vi "Spectrometer - Standalone.vi"() -> ()   [LabVIEW 2014]
uses:
  Laser Settings.ctl
  Laser.ctl
  Filter.ctl
  Grating Detector Settings.ctl
  Grating.ctl
  Detector.ctl
  Acquisition Settings.ctl
  support/Instrument Status.ctl
  Spectrometer Config.ctl
  Spectrometer Refnum.ctl
  Measurements/Plot Data/Optical Spectrum Plot Refnum.ctl
  support/User Event - Stop/User Event - Stop.lvlib
  support/Message Queue/Message Queue.lvlib
panel:
  out "Instrument Status":T1
  out "Status Log":string
  in  "Laser Settings":T2={"Laser Wavelength"=enum."633 nm", "Neutral Density Filter"=enum."1%"}
  in  "Spectrometer Settings":T5={"Confocal Hole Size (µm)"=150.0, "Grating"=1, "Detector"=enum."InGaAs Array"} {"Grating" items=["1800 l/mm", "150 l/mm"]}
  in  "Acquisition Settings":T8={"Acquisition Mode"=enum."Single Window", "Spectal Position (nm)"=480.0, "From (nm)"=632.0, "To (nm)"=1000.0, "Integration Time (s)"=3.0, "Number of Accumulations"=3, "AutoScanning"=FALSE, "Spike Removal"=FALSE}
  in  "Optical Spectrum":enum32{"Energy", "Wavelength", "Raman Shift"}(tab)
  out "Optical Spectrum vs Energy":cluster{"data":dbl[], "data":dbl[]}(graph)
  out "Optical Spectrum vs Wavelength":cluster{"data":dbl[], "data":dbl[]}(graph)
  out "Optical Spectrum vs Raman Shift":cluster{"data":dbl[], "data":dbl[]}(graph)
  in  "Optical Spectrometer - Save Measurement":bool
  in  "Optical Spectrometer - Measure":bool
  out "Detector Temperature":dbl
  in  "Use Labram HR":bool=TRUE
  out "Last Operation":string
  in  "Exit":bool
  # "LICENSED MATERIALS – PROPERTY OF IBM\nCopyright IBM Corp. 2016,\nALL RIGHTS RESERVED"
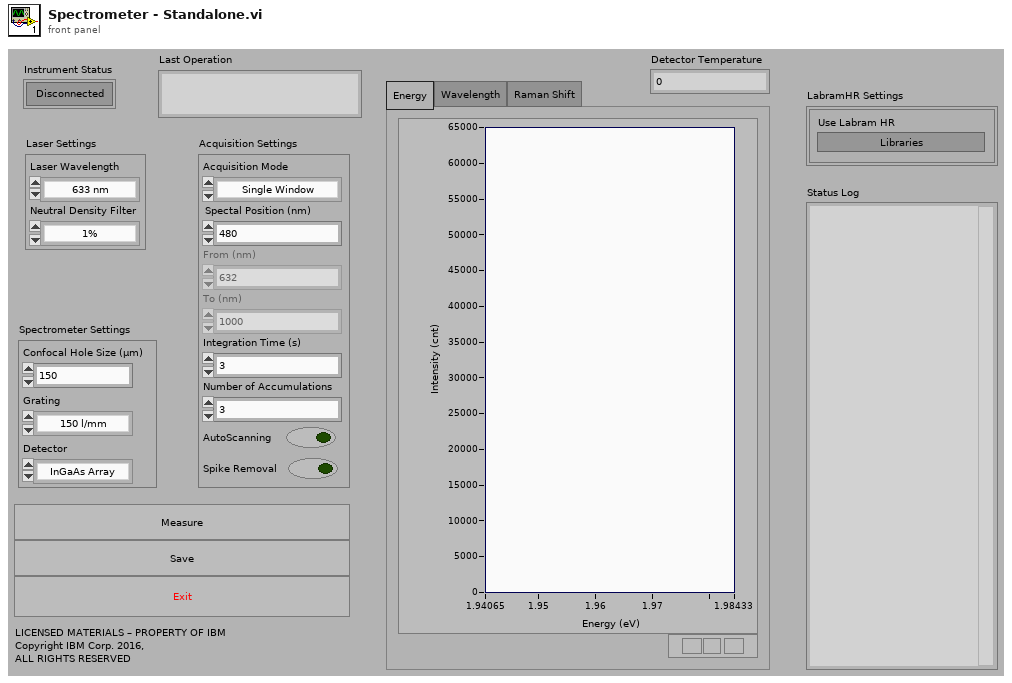
[diagram p1: front panel]
types:
  T1 = typedef "Instrument Status.ctl" = bool
  T2 = typedef "Laser Settings.ctl" = cluster{"Laser Wavelength":T3, "Neutral Density Filter":T4}
  T3 = typedef "Laser.ctl" = enum16{"633 nm", "784 nm", "532 nm", "365 nm"}
  T4 = typedef "Filter.ctl" = enum16{"100%", "50%", "25%", "10%", "1%", "0.1%", "0.01%"}
  T5 = typedef "Grating Detector Settings.ctl" = cluster{"Confocal Hole Size (µm)":dbl, "Grating":T6, "Detector":T7}
  T6 = typedef "Grating.ctl" = u16
  T7 = typedef "Detector.ctl" = enum16{"InGaAs Array", "Silicon CCD"}
  T8 = typedef "Acquisition Settings.ctl" = cluster{"Acquisition Mode":enum16{"Single Window", "Multi-Window"}, "Spectal Position (nm)":dbl, "From (nm)":dbl, "To (nm)":dbl, "Integration Time (s)":dbl, "Number of Accumulations":i32, "AutoScanning":bool, "Spike Removal":bool}
  T9 = typedef "Message Queue.lvlib/All Message Queues.ctl" = cluster{"Message Handler Loop":refnum<queue>, "Parameter Analyzer":refnum<queue>, "Switching Matrix":refnum<queue>, "Stress Control":refnum<queue>, "Optical Spectrometer":refnum<queue>, "Switches & Mirrors":refnum<queue>, "Camera":refnum<queue>, "XYZ Stage":refnum<queue>, "AutoFocus":refnum<queue>, "Optoelectronic":refnum<queue>, "Save Data":refnum<queue>, "Plot Data":refnum<queue>, "Instrument Sequence":refnum<queue>, "Strain Measurement":refnum<queue>}
  T10 = typedef "Notifiers.ctl" = cluster{"Message Handler Loop":T11, "Parameter Analyzer":T12, "Switching Matrix":T13, "Stress Control":T14, "Optical Spectrometer":T15, "Switches & Mirrors":T16, "Camera":T17, "XYZ Stage":T18, "AutoFocus":T19, "Optoelectronic":T20, "Save Data":T21, "Plot Data":T21, "Instrument Sequence":T22, "Strain Measurement":cluster{"Status":refnum<notifier>, "Exit":refnum<notifier>, "Ready":refnum<notifier>}}
  T11 = typedef "Message Handler Loop Notifiers.ctl" = cluster{"Status":refnum<notifier>, "Instrument Data":refnum<notifier>, "Exit":refnum<notifier>, "Ready":refnum<notifier>}
  T12 = typedef "Parameter Analyzer Notifiers.ctl" = cluster{"Status":refnum<notifier>, "Instrument Data":refnum<notifier>, "Measurement":refnum<notifier>, "Exit":refnum<notifier>, "Ready":refnum<notifier>}
  T13 = typedef "Switching Matrix Notifiers.ctl" = cluster{"Status":refnum<notifier>, "Instrument Data":refnum<notifier>, "Measurement":refnum<notifier>, "Exit":refnum<notifier>, "Ready":refnum<notifier>}
  T14 = typedef "StressControl Notifiers.ctl" = cluster{"Status":refnum<notifier>, "Instrument Data":refnum<notifier>, "Measurement":refnum<notifier>, "Exit":refnum<notifier>, "Ready":refnum<notifier>}
  T15 = typedef "Spectrometer Notifiers.ctl" = cluster{"Status":refnum<notifier>, "Instrument Data":refnum<notifier>, "Measurement":refnum<notifier>, "Exit":refnum<notifier>, "Ready":refnum<notifier>}
  T16 = typedef "SwitchesMirrors Notifiers.ctl" = cluster{"Status":refnum<notifier>, "Instrument Data":refnum<notifier>, "Exit":refnum<notifier>, "Ready":refnum<notifier>}
  T17 = typedef "Camera Notifiers.ctl" = cluster{"Status":refnum<notifier>, "Instrument Data":refnum<notifier>, "Measurement":refnum<notifier>, "Exit":refnum<notifier>, "Ready":refnum<notifier>}
  T18 = typedef "XYZ Notifications.ctl" = cluster{"Status":refnum<notifier>, "Instrument Data":refnum<notifier>, "Measurement":refnum<notifier>, "Exit":refnum<notifier>, "Ready":refnum<notifier>}
  T19 = typedef "Autofocus Notifiers.ctl" = cluster{"Status":refnum<notifier>, "Instrument Data":refnum<notifier>, "Measurement":refnum<notifier>, "Exit":refnum<notifier>, "Ready":refnum<notifier>}
  T20 = typedef "Optoelectronic Notifiers.ctl" = cluster{"Status":refnum<notifier>, "Instrument Data":refnum<notifier>, "Measurement":refnum<notifier>, "Exit":refnum<notifier>, "Ready":refnum<notifier>}
  T21 = typedef "SaveData Notifiers.ctl" = cluster{"Status":refnum<notifier>, "Exit":refnum<notifier>, "Ready":refnum<notifier>}
  T22 = typedef "Instrument Sequence Notifiers.ctl" = cluster{"Status":refnum<notifier>, "Instrument Data":refnum<notifier>, "Measurement":refnum<notifier>, "Exit":refnum<notifier>, "Ready":refnum<notifier>}
  T23 = typedef "Configuration.ctl" = cluster{"Parameter Analizer":T24, "Switching Matrix":T32, "Stress Control":T33, "Optical Spectrometer":T34, "Switches & Mirrors":T35, "Camera":T37, "XYZ Stage":T39, "AutoFocus":T43, "Sava Data":T46, "PlotData":T51, "Instrument Sequence":T57, "Strain Measurement":T58}
  T24 = typedef "Parameter Analyzer Config.ctl" = cluster{"Parameter Analyzer VISA Session":refnum<visa-resource-name>, "Sweeping Time Parameters":T25, "Acquisition Mode":enum32{"Sweeping Mode", "Sampling Mode"}, "Status Polling Time (ms)":u32, "Comment":string, "SMU 1 - Sweeping":T26, "SMU 2 - Sweeping":T26, "SMU 3 - Sweeping":T26, "SMU 4 - Sweeping":T26, "Sweep Spacing":T27, "Range":T28, "SMU1 - Sampling":T29, "SMU2 - Sampling":T29, "SMU3 - Sampling":T29, "SMU4 - Sampling":T29, "Sampling Time Parameters":T30, "Stop Condition":T31}
  T25 = typedef "Parameter Analyzer Integration Parameters.ctl" = cluster{"Integration Time":u32, "Short Integration Time (s)":dbl, "Long Integration Time (s)":dbl, "Wait Time Parameter":dbl}
  T26 = typedef "Parameter Analyzer SMU Sweeping.ctl" = cluster{"Start / Offset":dbl, "Stop / Ratio":dbl, "Step \n(linear only)":dbl, "Compliance":dbl, "Power \nCompliance":dbl, "Mode":u32, "Function":i32, "Sweep Mode":bool}
  T27 = typedef "Parameter Analyzer Sweep Spacing.ctl" = u16
  T28 = typedef "Parameter Analyzer SMU Range.ctl" = u16
  T29 = typedef "Parameter Analyzer SMU Sampling.ctl" = cluster{"Source":dbl, "Compliance":dbl, "Mode":u32, "Function":bool}
  T30 = typedef "Parameter Analyzer Sampling Parameters.ctl" = cluster{"Initial Interval (s)":dbl, "Number of Samples":i32, "Total Sampling Time (s)":dbl, "Hold Time (s)":dbl, "Sampling Mode":i32, "Sampling Time":i32}
  T31 = typedef "Parameter Analyzer Stop Sampling Conditions.ctl" = cluster{"Enable Delay (s)":dbl, "Name":string, "Threshold":dbl, "num. of events":i32, "Event":i32, "Stop Condition Enable":bool}
  T32 = typedef "Switching Matrix Config.ctl" = cluster{"Switching Matrix VISA Session":refnum<visa-resource-name>, "Connections":cluster{"Connections":bool[], "Connection Type":enum16{"Disconnected", "Make - Break", "Break - Make"}}[]}
  T33 = typedef "StressControl Config.ctl" = cluster{"Stress Control VISA Session":refnum<visa-resource-name>, "Axis":i32, "Motion":u16, "Destination (°)":dbl, "Speed (°/s)":dbl, "Position (°)":dbl}
  T34 = typedef "Spectrometer Config.ctl" = cluster{"Laser Settings":T2, "Spectrometer Settings":T5, "Acquisition Settings":T8, "Path":path}
  T35 = typedef "SwitchesMirrors Config.ctl" = cluster{"Relay VISA Session":refnum<visa-resource-name>, "Switches":T36, "Delays (ms)":cluster{"Laser":u32, "Video":u32}}
  T36 = typedef "SwitchesMirrors Status.ctl" = cluster{"Laser":bool, "Video":bool}
  T37 = typedef "Camera Config.ctl" = cluster{"Settings":T38}
  T38 = typedef "Camera Settings.ctl" = cluster{"Pixel clock":i32, "Frame rate":dbl, "Exposure time":dbl, "Master Gain":i32, "Red Gain":i32, "Green Gain":i32, "Blue Gain":i32, "Auto Gain":bool, "White-balance":bool, "Color Correction":bool}
  T39 = typedef "XYZ Config.ctl" = cluster{"Connection Settings":T40, "Manual Control":T41, "Coordinate Control":T42}
  T40 = typedef "XYZ Connection Settings.ctl" = cluster{"Tango VISA":refnum<visa-resource-name>, "Baudrate":i32, "Show Protocol?":bool}
  T41 = typedef "XYZ Stage Control.ctl" = cluster{"North":bool, "South":bool, "West":bool, "East":bool, "Up":bool, "Down":bool, "Stop":bool, "XY Step":dbl, "Z step":dbl}
  T42 = typedef "XYZ Coordinate Control.ctl" = cluster{"Motion Mode":enum16{"Absolute", "Relative"}, "Destination [mm]":dbl[]}
  T43 = typedef "AutoFocus Config.ctl" = cluster{"Matching Criteria":cluster{"Minimum Score":sgl, "Color Score Weight":sgl, "Minimum Contrast":i32, "Match Mode":u32, "Match Feature Mode":u32, "Subpixel Accuracy":bool, "Color Sensitivity":u32, "Search Strategy":u32}, "Z Scan Parameters":T44, "Displacement":dbl, "Transformation Matrix":T45}
  T44 = typedef "ZScan.ctl" = cluster{"Z Range":ext, "Resolution":dbl, "Initial Direction":enum16{"Up", "Down"}, "Focus Threshold":dbl, "Ascent Constant":dbl}
  T45 = typedef "NI_Matrix.lvlib/RealMatrix.ctl" = dbl[][]
  T46 = typedef "SaveData Config.ctl" = cluster{"Workspace Info":T47, "Instrument Configuration":T48, "Stress Motor Position":dbl, "Electrical Measurement":cluster{"Sequence":dbl[], "V1":dbl[], "V2":dbl[], "V3":dbl[], "V4":dbl[], "I1":dbl[], "I2":dbl[], "I3":dbl[], "I4":dbl[]}, "Optical Spectrum":T50}
  T47 = typedef "SaveData Workspace Info.ctl" = cluster{"Device Name":string, "Device Info":string, "Path":path}
  T48 = typedef "SaveData Instrument Configuration.ctl" = cluster{"Instrument":T49, "Configuration":string}
  T49 = typedef "Instrument List.ctl" = enum32{"Unknown Instrument", "Switching Matrix", "Parameter Analyzer", "Optical Spectrometer", "Optoelectronic", "Autofocus"}
  T50 = typedef "Spectral Data.ctl" = cluster{"Intensity":dbl[], "Wavelength":dbl[], "Energy":dbl[], "Raman Shift":dbl[], "Detector Temperature":dbl}
  T51 = typedef "PlotData Config.ctl" = cluster{"Sliders":cluster{"Strain Sequence":i32, "Instrument Sequence":i32}, "Measurement":T52, "Instrument Steps":T55, "Strain Points":dbl[]}
  T52 = typedef "Measurement.ctl" = cluster{"Which Instrument?":T53, "Electrical Measurement":T54, "Measurement Mode":enum16{"Sweeping Mode", "Sampling Mode"}, "Optical Spectrum":T50}
  T53 = typedef "WhichInstrument.ctl" = enum16{"No Plot", "Spectrometer", "Parameter Analyzer", "Optoelectronic"}
  T54 = typedef "Electrical Data.ctl" = cluster{"Sequence":dbl[], "V1":dbl[], "V2":dbl[], "V3":dbl[], "V4":dbl[], "I1":dbl[], "I2":dbl[], "I3":dbl[], "I4":dbl[]}
  T55 = typedef "Instrument Steps.ctl" = cluster{"Action":T56, "Configuration":variant, "Instrument":T49, "Status":enum8{"False", "True", "Mixed"}}[]
  T56 = typedef "Action.ctl" = enum32{"Configure", "Measure"}
  T57 = typedef "Instrument Sequence Config.ctl" = cluster{"Caller VI":enum16{"User", "Stress Measurement VI"}}
  T58 = typedef "Strain Measurement Config.ctl" = cluster{"Stress Sequence ":cluster{"Max Motor Position":ext, "# Intermediate Points":u32, "Initial Direction":enum16{"Tension", "Compression"}}, "Track?":bool}
  T59 = typedef "Spectrometer Refnum.ctl" = cluster{"Instrument Status":refnum<vi>, "Optical Spectrum Plot":T60, "Laser":refnum<vi>, "Filter":refnum<vi>, "Laser ON?":refnum<vi>, "Hole":refnum<vi>, "Grating":refnum<vi>, "Detector":refnum<vi>, "Acquisition Mode":refnum<vi>, "Spectal Position":refnum<vi>, "From":refnum<vi>, "To":refnum<vi>, "Integration Time":refnum<vi>, "Accumulations":refnum<vi>, "AutoScanning":refnum<vi>, "Spike Removal":refnum<vi>, "Acquisition Mode Panel":refnum<vi>}
  T60 = typedef "Optical Spectrum Plot Refnum.ctl" = cluster{"Plot List":refnum<vi>, "Optical Spectrum vs Energy":refnum<vi>, "Optical Spectrum vs Wavelength":refnum<vi>, "Optical Spectrum vs Raman Shift":refnum<vi>, "Detector Temperature":refnum<vi>}
  T61 = enum32{"invalid app kind", "Development System", "Run Time System", "Student Edition", "Embedded LabVIEW", "Evaluation", "Custom"}
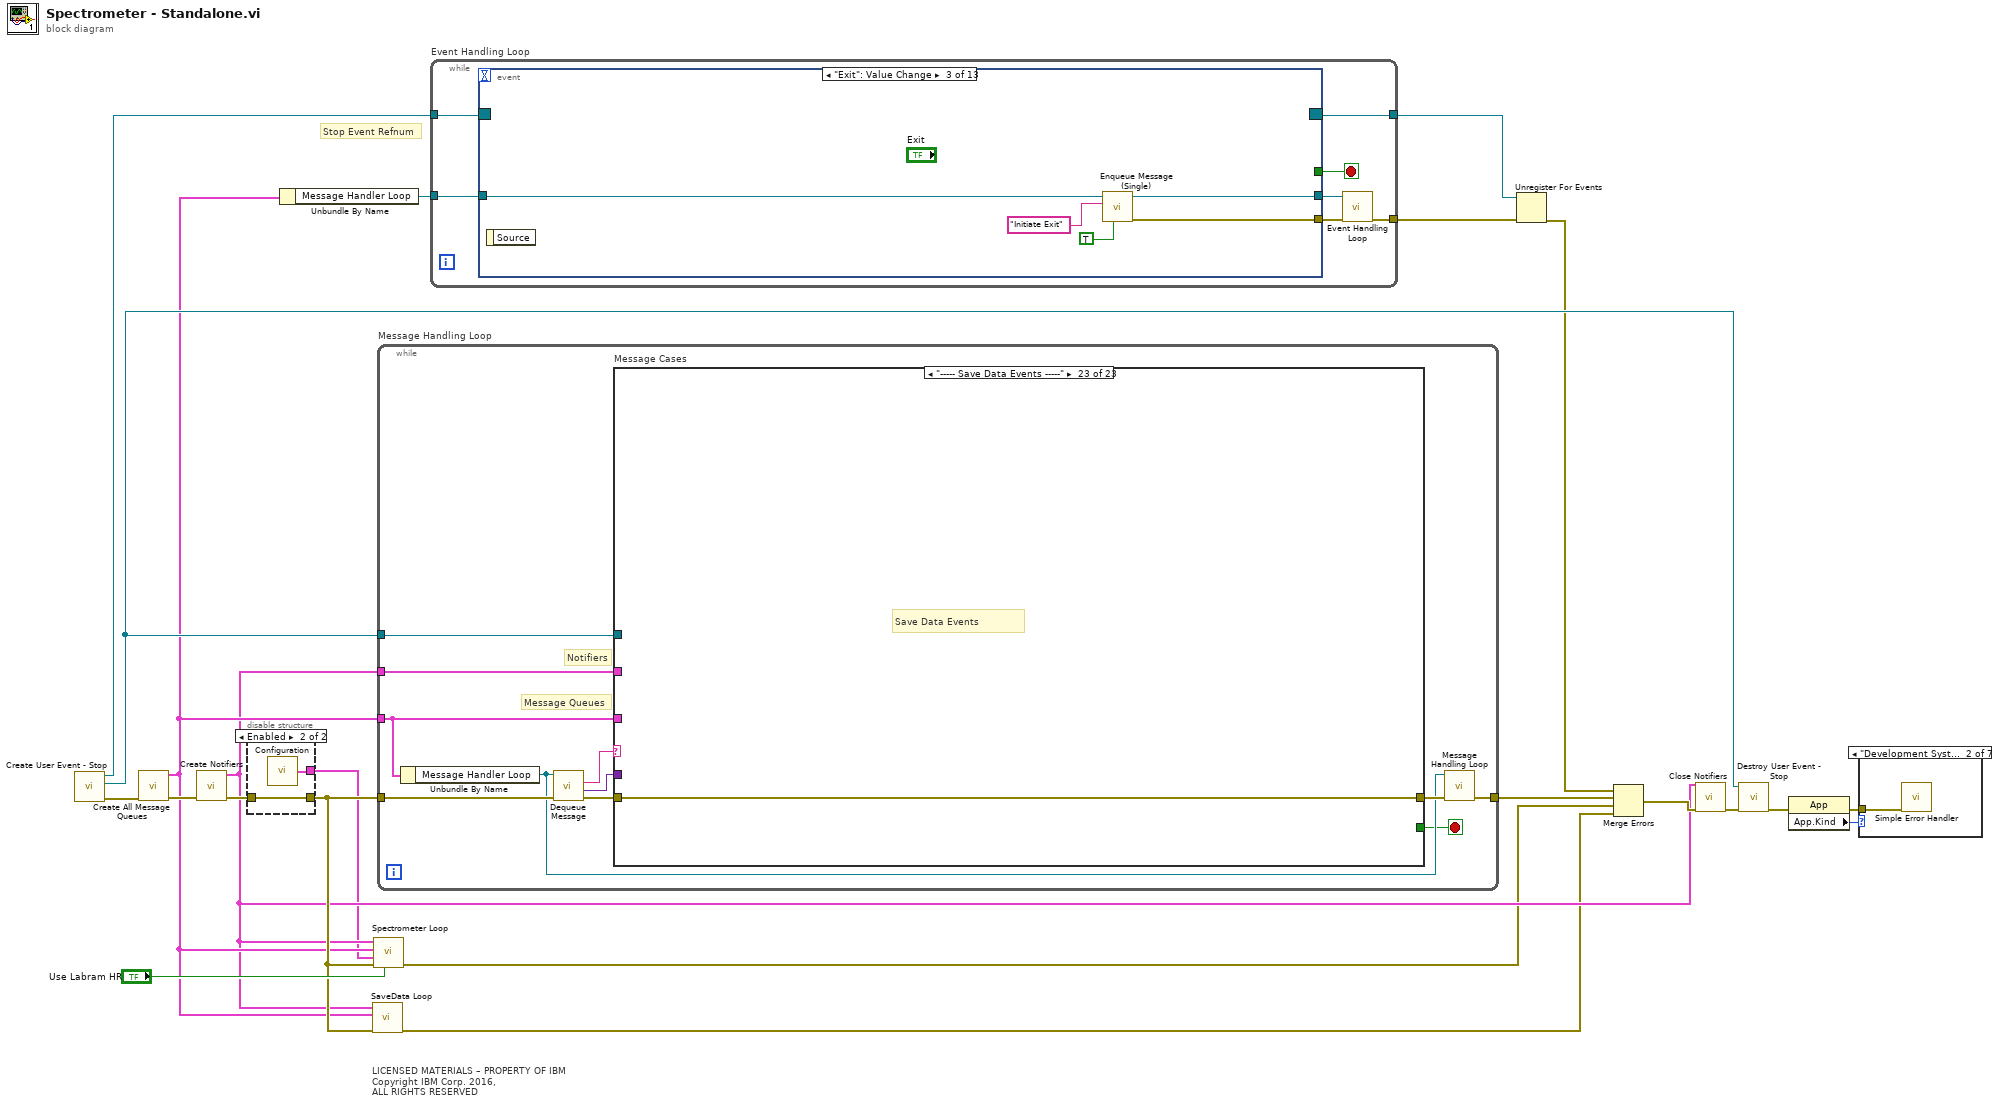
[diagram p0: block diagram]
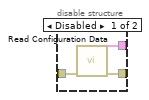
[diagram p2: hidden frame]
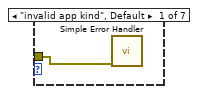
[diagram p3: hidden frame]
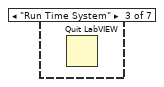
[diagram p4: hidden frame]
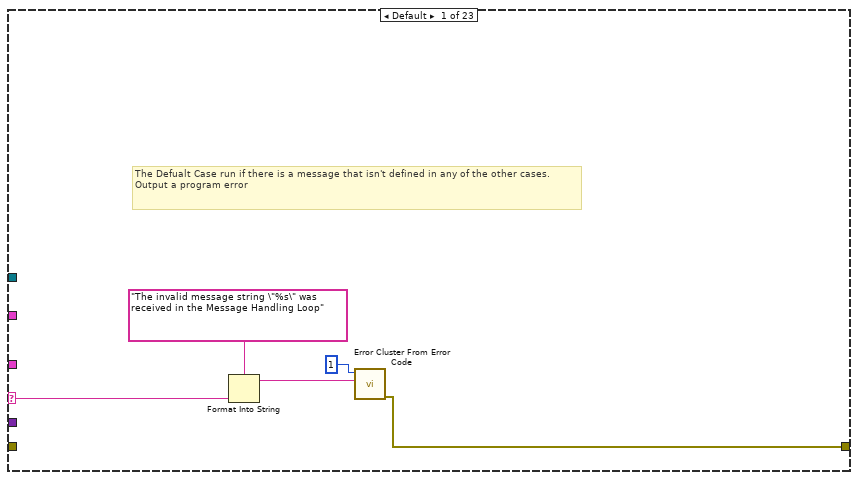
[diagram p9: hidden frame]
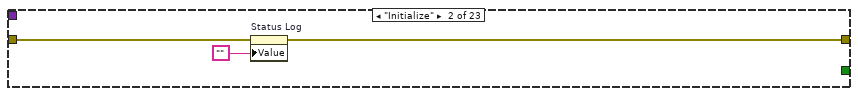
[diagram p10: hidden frame]
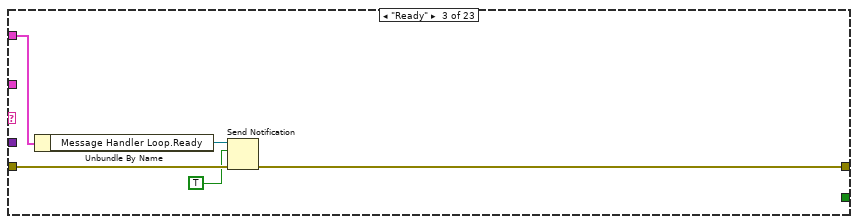
[diagram p11: hidden frame]
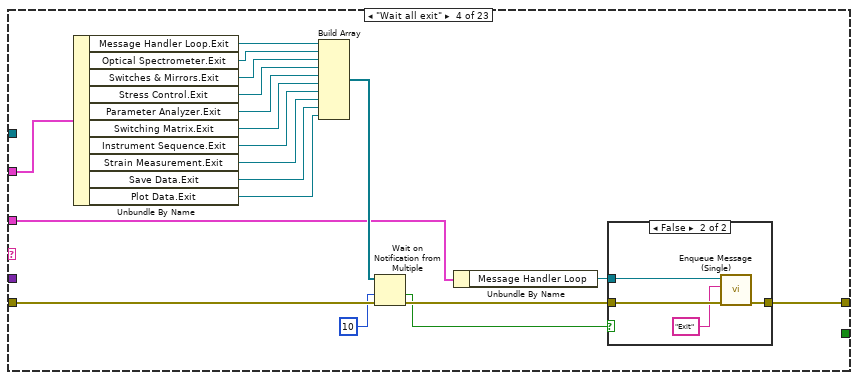
[diagram p12: hidden frame]
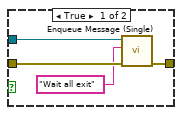
[diagram p13: hidden frame]
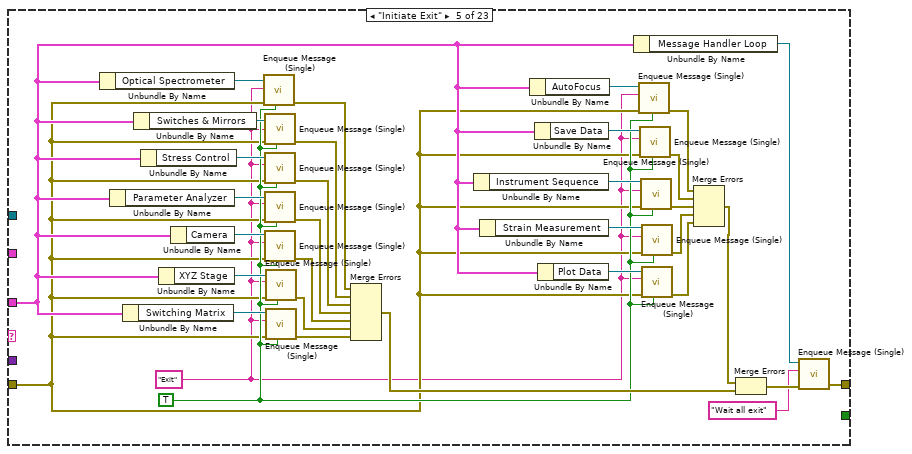
[diagram p14: hidden frame]
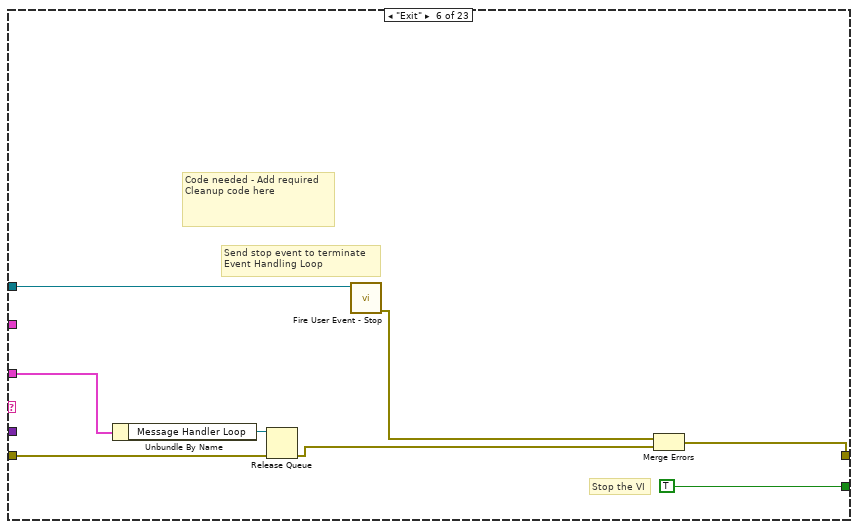
[diagram p15: hidden frame]
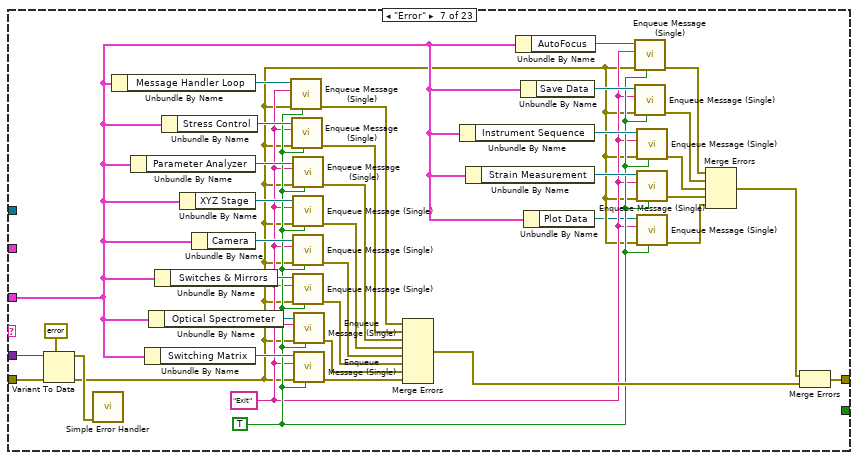
[diagram p16: hidden frame]
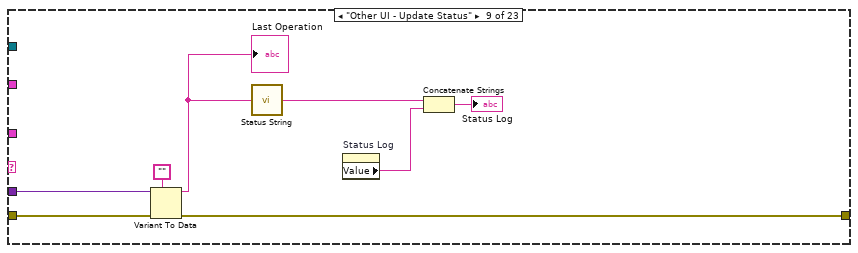
[diagram p18: hidden frame]
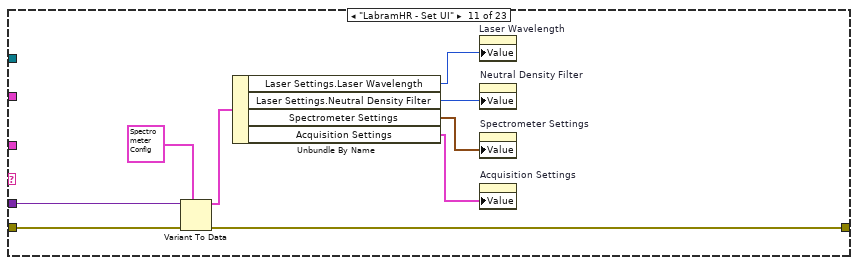
[diagram p20: hidden frame]
diagram:
  # "LICENSED MATERIALS – PROPERTY OF IBM\nCopyright IBM Corp. 2016,\nALL RIGHTS RESERVED"
  # "Stop Event Refnum"
  n1 = call "Create User Event - Stop.vi"() -> ("error out"=w12:errorcluster, "User Event - Stop"=w15:refnum<user-event>, "Stop Event Registration Refnum"=w22:refnum<event-registration>)  [unwired: 1 in, 8 out]
  n2 = call "Create All Message Queues.vi"("error in (no error)"=w12) -> ("error out"=w11:errorcluster, "Message Queues out"=w7:T9)  [unwired: 9 out]
  n3 = call "Create Notifiers.vi"("error in"=w11) -> ("error out"=w10:errorcluster, "Notifiers"=w6:T10)  [unwired: 9 out]
  n4 = disable-structure shown="Enabled" {
    disable-tunnel: w10 -> [w25 w27]
    disable-tunnel: [w24 w27] -> w8
    disable-tunnel: [w23 w26] -> w2
    frame Disabled {
      n5 = call "Read Configuration Data.vi"("error in"=w25) -> ("error out"=w24:errorcluster, "System Configuration"=w23:T23)  [unwired: 9 out]
    }
    frame Enabled {
      n6 = call "Configuration.vi"() -> ("IBM OptoElectroMechanics Configuration"=w26:T23)
    }
  }
  n7 = Unbundle By Name(w7) -> ("Message Handler Loop"=w20:refnum<queue>)
  n8 = call "SaveData Loop.vi"("error in"=w8, "Message Queues out"=w7, "Notifiers"=w6) -> ("error out"=w1:errorcluster)  [unwired: 1 in, 7 out]
  n9 = call "Spectrometer Loop.vi"("Used functions"="Use Labram HR", "error in"=w8, "Configuration"=w2, "Message Queues out"=w7, "Notifiers"=w6) -> ("error out"=w3:errorcluster)  [unwired: 6 out]
  n10 = while "Message Handling Loop" {
    tunnel: w8 -> [w38]
    tunnel: [w35] -> w4
    tunnel: w7 -> [w29]
    tunnel: w15 -> [w31]
    tunnel: w6 -> [w28]
    stop <- w30 stop-if-true
    # "Notifiers"
    # "Message Queues"
    n11 = Unbundle By Name(w29) -> ("Message Handler Loop"=w34:refnum<queue>)
    n12 = call "Dequeue Message.vi"("error in (no error)"=w38, "Message Queue"=w34) -> ("error out"=w37:errorcluster, "Message Data"=w32:variant, "Message"=w33:string)  [unwired: 7 out]
    n13 = case "Message Cases" shown="\"----- Save Data Events -----\"" w33 {
      selector: w33 -> [w43 _ _ _ _ _ _ _ _ _ _ _ _ _ _ _ _ _ _ _ _ _ _]
      tunnel: w37 -> [_ w45 w50 w69 w82 w119 w146 w158 w166 w167 w175 w198 w208 w223 w234 w245 w256 w267 w278 w282 w287 w289 w294]
      tunnel: [w39 w44 w51 w58 w98 w120 w155 w158 w163 w167 w174 w198 w206 w219 w230 w242 w253 w263 w276 w279 w284 w291 w294] -> w36
      tunnel: w32 -> [_ _ _ _ _ _ w157 _ w165 _ w169 _ w212 w222 w233 w244 w255 w266 w277 _ _ _ _]
      tunnel: w31 -> [_ _ _ _ _ w117 _ _ _ _ _ _ _ _ _ _ _ _ _ _ _ _ _]
      tunnel: [_ _ _ _ _ TRUE _ _ _ _ _ _ _ _ _ _ _ _ _ _ _ _ _] -> w30
      tunnel: w29 -> [_ _ _ w57 w85 w114 w127 _ _ _ _ w201 w211 w218 w227 w240 w251 w260 w272 w280 w285 w293 _]
      tunnel: w28 -> [_ _ w49 w70 _ _ _ _ _ _ _ _ _ _ _ _ _ _ _ _ _ _ _]
      frame Default {
        # "The Defualt Case run if there is a message that isn't defined in any of the other cases.\nOutput a program error"
        n14 = Format Into String(format string="The invalid message string \"%s\" was  received in the Message Handling Loop", w43) -> (resulting string=w41:string)  [unwired: 2 in, 1 out]
        n15 = call <vilib>:"Error Cluster From Error Code.vi"("error message (\"\")"=w41, "error code (0)"=1) -> ("error out"=w39:errorcluster)  [unwired: 2 in, 5 out]
      }
      frame "Initialize" {
        n16 = property on="Status Log" class="Str"(error in=w45, "Value"="") -> (error out=w44:errorcluster)  [unwired: 1 in, 1 out]
      }
      frame "Ready" {
        n17 = Unbundle By Name(w49) -> ("Message Handler Loop.Ready"=w48:refnum<notifier>)
        n18 = Send Notification(notification=TRUE, notifier=w48, error in (no error)=w50) -> (error out=w51:errorcluster)  [unwired: 1 out]
      }
      frame "Wait all exit" {
        n19 = Unbundle By Name(w70) -> ("Message Handler Loop.Exit"=w67:refnum<notifier>, "Optical Spectrometer.Exit"=w66:refnum<notifier>, "Switches & Mirrors.Exit"=w65:refnum<notifier>, "Stress Control.Exit"=w64:refnum<notifier>, "Parameter Analyzer.Exit"=w63:refnum<notifier>, "Switching Matrix.Exit"=w62:refnum<notifier>, "Instrument Sequence.Exit"=w55:refnum<notifier>, "Strain Measurement.Exit"=w54:refnum<notifier>, "Save Data.Exit"=w53:refnum<notifier>, "Plot Data.Exit"=w52:refnum<notifier>)
        n20 = Build Array(w67, w66, w65, w64, w63, w62, w55, w54, w53, w52) -> (w61:refnum<notifier>[])
        n21 = Wait on Notification from Multiple(0:w61, 2:10 ("timeout in ms (-1)"), 3:w69) -> (10:w56:bool, 11:w59:errorcluster)  [unwired: 3 out]
        n22 = Unbundle By Name(w57) -> ("Message Handler Loop"=w60:refnum<queue>)
        n23 = case shown="False" w56 {
          tunnel: w60 -> [w74 w78]
          tunnel: w59 -> [w73 w77]
          tunnel: [w72 w76] -> w58
          frame True {
            n24 = call "Enqueue Message (Single).vi"("error in (no error)"=w73, "Message"="Wait all exit", "Message Queue"=w74) -> ("error out"=w72:errorcluster)  [unwired: 1 in, 7 out]
          }
          frame False {
            n25 = call "Enqueue Message (Single).vi"("error in (no error)"=w77, "Message"="Exit", "Message Queue"=w78) -> ("error out"=w76:errorcluster)  [unwired: 1 in, 7 out]
          }
        }
      }
      frame "Initiate Exit" {
        w83 = TRUE ("Priority Message? (F)")
        w80 = "Exit" ("Message")
        n26 = Unbundle By Name(w85) -> ("Optical Spectrometer"=w102:refnum<queue>)
        n27 = Unbundle By Name(w85) -> ("Parameter Analyzer"=w99:refnum<queue>)
        n28 = Unbundle By Name(w85) -> ("Switching Matrix"=w94:refnum<queue>)
        n29 = Unbundle By Name(w85) -> ("Switches & Mirrors"=w101:refnum<queue>)
        n30 = Unbundle By Name(w85) -> ("Stress Control"=w100:refnum<queue>)
        n31 = Unbundle By Name(w85) -> ("XYZ Stage"=w112:refnum<queue>)
        n32 = Unbundle By Name(w85) -> ("Camera"=w103:refnum<queue>)
        n33 = call "Enqueue Message (Single).vi"("Priority Message? (F)"=w83, "error in (no error)"=w82, "Message"=w80, "Message Queue"=w102) -> ("error out"=w104:errorcluster)  [unwired: 1 in, 6 out]
        n34 = call "Enqueue Message (Single).vi"("Priority Message? (F)"=w83, "error in (no error)"=w82, "Message"=w80, "Message Queue"=w101) -> ("error out"=w105:errorcluster)  [unwired: 1 in, 6 out]
        n35 = call "Enqueue Message (Single).vi"("Priority Message? (F)"=w83, "error in (no error)"=w82, "Message"=w80, "Message Queue"=w100) -> ("error out"=w106:errorcluster)  [unwired: 1 in, 6 out]
        n36 = call "Enqueue Message (Single).vi"("Priority Message? (F)"=w83, "error in (no error)"=w82, "Message"=w80, "Message Queue"=w99) -> ("error out"=w107:errorcluster)  [unwired: 1 in, 6 out]
        n37 = call "Enqueue Message (Single).vi"("Priority Message? (F)"=w83, "error in (no error)"=w82, "Message"=w80, "Message Queue"=w103) -> ("error out"=w108:errorcluster)  [unwired: 1 in, 6 out]
        n38 = call "Enqueue Message (Single).vi"("Priority Message? (F)"=w83, "error in (no error)"=w82, "Message"=w80, "Message Queue"=w112) -> ("error out"=w109:errorcluster)  [unwired: 1 in, 6 out]
        n39 = call "Enqueue Message (Single).vi"("Priority Message? (F)"=w83, "error in (no error)"=w82, "Message"=w80, "Message Queue"=w94) -> ("error out"=w110:errorcluster)  [unwired: 1 in, 6 out]
        n40 = Merge Errors(w104, w105, w106, w107, w108, w109, w110) -> (w111:errorcluster)
        n41 = Unbundle By Name(w85) -> ("Instrument Sequence"=w91:refnum<queue>)
        n42 = Unbundle By Name(w85) -> ("Strain Measurement"=w87:refnum<queue>)
        n43 = Unbundle By Name(w85) -> ("AutoFocus"=w93:refnum<queue>)
        n44 = Unbundle By Name(w85) -> ("Save Data"=w92:refnum<queue>)
        n45 = Unbundle By Name(w85) -> ("Plot Data"=w84:refnum<queue>)
        n46 = Unbundle By Name(w85) -> ("Message Handler Loop"=w96:refnum<queue>)
        n47 = call "Enqueue Message (Single).vi"("Priority Message? (F)"=w83, "error in (no error)"=w82, "Message"=w80, "Message Queue"=w93) -> ("error out"=w90:errorcluster)  [unwired: 1 in, 6 out]
        n48 = call "Enqueue Message (Single).vi"("Priority Message? (F)"=w83, "error in (no error)"=w82, "Message"=w80, "Message Queue"=w92) -> ("error out"=w89:errorcluster)  [unwired: 1 in, 6 out]
        n49 = call "Enqueue Message (Single).vi"("Priority Message? (F)"=w83, "error in (no error)"=w82, "Message"=w80, "Message Queue"=w91) -> ("error out"=w88:errorcluster)  [unwired: 1 in, 6 out]
        n50 = call "Enqueue Message (Single).vi"("Priority Message? (F)"=w83, "error in (no error)"=w82, "Message"=w80, "Message Queue"=w87) -> ("error out"=w86:errorcluster)  [unwired: 1 in, 6 out]
        n51 = call "Enqueue Message (Single).vi"("Priority Message? (F)"=w83, "error in (no error)"=w82, "Message"=w80, "Message Queue"=w84) -> ("error out"=w81:errorcluster)  [unwired: 1 in, 6 out]
        n52 = Merge Errors(w90, w89, w88, w86, w81) -> (w79:errorcluster)
        n53 = Merge Errors(w79, w111) -> (w97:errorcluster)
        n54 = call "Enqueue Message (Single).vi"("error in (no error)"=w97, "Message"="Wait all exit", "Message Queue"=w96) -> ("error out"=w98:errorcluster)  [unwired: 1 in, 7 out]
      }
      frame "Exit" {
        # "Send stop event to terminate \nEvent Handling Loop"
        # "Stop the VI"
        # "Code needed - Add required Cleanup code here"
        n55 = Unbundle By Name(w114) -> ("Message Handler Loop"=w113:refnum<queue>)
        n56 = Release Queue(queue=w113, error in (no error)=w119) -> (error out=w118:errorcluster)  [unwired: 3 out]
        n57 = call "Fire User Event - Stop.vi"("User Event - Stop"=w117) -> ("error out"=w116:errorcluster)  [unwired: 1 in, 9 out]
        n58 = Merge Errors(w116, w118) -> (w120:errorcluster)
      }
      frame "Error" {
        w126 = TRUE ("Priority Message? (F)")
        w125 = "Exit" ("Message")
        n59 = Variant To Data(error in=w146, type=errorcluster {"status"=FALSE, "code"=0, "source"=""} ("error out"), Variant=w157) -> (data=w154:errorcluster, error out=w123:errorcluster)
        n60 = call <vilib>:"Simple Error Handler.vi"("error in (no error)"=w154) -> ()  [unwired: 1 in, 8 out]
        n61 = Unbundle By Name(w127) -> ("Message Handler Loop"=w137:refnum<queue>)
        n62 = Unbundle By Name(w127) -> ("Parameter Analyzer"=w152:refnum<queue>)
        n63 = Unbundle By Name(w127) -> ("Switching Matrix"=w147:refnum<queue>)
        n64 = Unbundle By Name(w127) -> ("Optical Spectrometer"=w148:refnum<queue>)
        n65 = Unbundle By Name(w127) -> ("Switches & Mirrors"=w138:refnum<queue>)
        n66 = Unbundle By Name(w127) -> ("Stress Control"=w151:refnum<queue>)
        n67 = Unbundle By Name(w127) -> ("XYZ Stage"=w153:refnum<queue>)
        n68 = Unbundle By Name(w127) -> ("Camera"=w139:refnum<queue>)
        n69 = call "Enqueue Message (Single).vi"("Priority Message? (F)"=w126, "error in (no error)"=w123, "Message"=w125, "Message Queue"=w137) -> ("error out"=w136:errorcluster)  [unwired: 1 in, 6 out]
        n70 = call "Enqueue Message (Single).vi"("Priority Message? (F)"=w126, "error in (no error)"=w123, "Message"=w125, "Message Queue"=w151) -> ("error out"=w145:errorcluster)  [unwired: 1 in, 6 out]
        n71 = call "Enqueue Message (Single).vi"("Priority Message? (F)"=w126, "error in (no error)"=w123, "Message"=w125, "Message Queue"=w152) -> ("error out"=w144:errorcluster)  [unwired: 1 in, 6 out]
        n72 = call "Enqueue Message (Single).vi"("Priority Message? (F)"=w126, "error in (no error)"=w123, "Message"=w125, "Message Queue"=w153) -> ("error out"=w143:errorcluster)  [unwired: 1 in, 6 out]
        n73 = call "Enqueue Message (Single).vi"("Priority Message? (F)"=w126, "error in (no error)"=w123, "Message"=w125, "Message Queue"=w139) -> ("error out"=w142:errorcluster)  [unwired: 1 in, 6 out]
        n74 = call "Enqueue Message (Single).vi"("Priority Message? (F)"=w126, "error in (no error)"=w123, "Message"=w125, "Message Queue"=w138) -> ("error out"=w141:errorcluster)  [unwired: 1 in, 6 out]
        n75 = call "Enqueue Message (Single).vi"("Priority Message? (F)"=w126, "error in (no error)"=w123, "Message"=w125, "Message Queue"=w148) -> ("error out"=w150:errorcluster)  [unwired: 1 in, 6 out]
        n76 = call "Enqueue Message (Single).vi"("Priority Message? (F)"=w126, "error in (no error)"=w123, "Message"=w125, "Message Queue"=w147) -> ("error out"=w149:errorcluster)  [unwired: 1 in, 6 out]
        n77 = Merge Errors(w136, w145, w144, w143, w142, w141, w150, w149) -> (w140:errorcluster)
        n78 = Unbundle By Name(w127) -> ("Instrument Sequence"=w133:refnum<queue>)
        n79 = Unbundle By Name(w127) -> ("Strain Measurement"=w129:refnum<queue>)
        n80 = Unbundle By Name(w127) -> ("AutoFocus"=w135:refnum<queue>)
        n81 = Unbundle By Name(w127) -> ("Save Data"=w134:refnum<queue>)
        n82 = Unbundle By Name(w127) -> ("Plot Data"=w122:refnum<queue>)
        n83 = call "Enqueue Message (Single).vi"("Priority Message? (F)"=w126, "error in (no error)"=w123, "Message"=w125, "Message Queue"=w135) -> ("error out"=w130:errorcluster)  [unwired: 1 in, 6 out]
        n84 = call "Enqueue Message (Single).vi"("Priority Message? (F)"=w126, "error in (no error)"=w123, "Message"=w125, "Message Queue"=w134) -> ("error out"=w131:errorcluster)  [unwired: 1 in, 6 out]
        n85 = call "Enqueue Message (Single).vi"("Priority Message? (F)"=w126, "error in (no error)"=w123, "Message"=w125, "Message Queue"=w133) -> ("error out"=w132:errorcluster)  [unwired: 1 in, 6 out]
        n86 = call "Enqueue Message (Single).vi"("Priority Message? (F)"=w126, "error in (no error)"=w123, "Message"=w125, "Message Queue"=w129) -> ("error out"=w128:errorcluster)  [unwired: 1 in, 6 out]
        n87 = call "Enqueue Message (Single).vi"("Priority Message? (F)"=w126, "error in (no error)"=w123, "Message"=w125, "Message Queue"=w122) -> ("error out"=w124:errorcluster)  [unwired: 1 in, 6 out]
        n88 = Merge Errors(w130, w131, w132, w128, w124) -> (w121:errorcluster)
        n89 = Merge Errors(w121, w140) -> (w155:errorcluster)
      }
      frame "----- Other UI Events -----" {
        # "Other UI Events"
      }
      frame "Other UI - Update Status" {
        n90 = Variant To Data(error in=w166, type="", Variant=w165) -> (data=w159:string, error out=w163:errorcluster)
        "Last Operation" <- w159
        n91 = call "Status String.vi"("Message"=w159) -> ("Status String"=w162:string)
        n92 = property on="Status Log" class="Str"() -> ("Value"=w160:string)  [unwired: 2 in, 2 out]
        n93 = Concatenate Strings(w162, w160) -> (→"Status Log":string)
      }
      frame "----- Spectrometer Events -----" {
        # "Spectrometer Events"
      }
      frame "LabramHR - Set UI" {
        n94 = Variant To Data(error in=w175, type=T34 {"Laser Settings"={"Laser Wavelength"=enum."633 nm", "Neutral Density Filter"=enum."1%"}, "Spectrometer Settings"={"Confocal Hole Size (µm)"=150.0, "Grating"=1, "Detector"=enum."InGaAs Array"}, "Acquisition Settings"={"Acquisition Mode"=enum."Single Window", "Spectal Position (nm)"=480.0, "From (nm)"=632.0, "To (nm)"=1000.0, "Integration Time (s)"=3.0, "Number of Accumulations"=3, "AutoScanning"=FALSE, "Spike Removal"=FALSE}, "Path"=path ""} ("LabramHR"), Variant=w169) -> (data=w176:T34, error out=w174:errorcluster)
        n95 = Unbundle By Name(w176) -> ("Laser Settings.Laser Wavelength"=w171:T3, "Laser Settings.Neutral Density Filter"=w170:T4, "Spectrometer Settings"=w173:T5, "Acquisition Settings"=w172:T8)
        n96 = property on="Laser Wavelength" class="Enum (strict)"("Value"=w171) -> ()  [unwired: 2 in, 2 out]
        n97 = property on="Neutral Density Filter" class="Enum (strict)"("Value"=w170) -> ()  [unwired: 2 in, 2 out]
        n98 = property on="Spectrometer Settings" class="Clust (strict)"("Value"=w173) -> ()  [unwired: 2 in, 2 out]
        n99 = property on="Acquisition Settings" class="Clust (strict)"("Value"=w172) -> ()  [unwired: 2 in, 2 out]
      }
      frame "LabramHR - Update Refnums" {
        n100 = control-ref of="Optical Spectrum"() -> (w196:refnum<vi>)
        n101 = control-ref of="Optical Spectrum vs Energy"() -> (w195:refnum<vi>)
        n102 = control-ref of="Optical Spectrum vs Wavelength"() -> (w194:refnum<vi>)
        n103 = control-ref of="Optical Spectrum vs Raman Shift"() -> (w193:refnum<vi>)
        n104 = control-ref of="AutoScanning"() -> (w184:refnum<vi>)
        n105 = control-ref of="Spike Removal"() -> (w185:refnum<vi>)
        n106 = control-ref of="Detector Temperature"() -> (w179:refnum<vi>)
        n107 = control-ref of="Confocal Hole Size (µm)"() -> (w190:refnum<vi>)
        n108 = control-ref of="Spectal Position (nm)"() -> (w180:refnum<vi>)
        n109 = control-ref of="From (nm)"() -> (w186:refnum<vi>)
        n110 = control-ref of="To (nm)"() -> (w181:refnum<vi>)
        n111 = control-ref of="Integration Time (s)"() -> (w182:refnum<vi>)
        n112 = control-ref of="Number of Accumulations"() -> (w183:refnum<vi>)
        n113 = control-ref of="Laser Wavelength"() -> (w192:refnum<vi>)
        n114 = control-ref of="Neutral Density Filter"() -> (w191:refnum<vi>)
        n115 = control-ref of="Detector"() -> (w188:refnum<vi>)
        n116 = control-ref of="Acquisition Mode"() -> (w187:refnum<vi>)
        n117 = control-ref of="Grating"() -> (w189:refnum<vi>)
        n118 = control-ref of="Instrument Status"() -> (w177:refnum<vi>)
        n119 = Bundle By Name(cluster=T59 {"Instrument Status"=refnum, "Optical Spectrum Plot"={"Plot List"=refnum, "Optical Spectrum vs Energy"=refnum, "Optical Spectrum vs Wavelength"=refnum, "Optical Spectrum vs Raman Shift"=refnum, "Detector Temperature"=refnum}, "Laser"=refnum, "Filter"=refnum, "Laser ON?"=refnum, "Hole"=refnum, "Grating"=refnum, "Detector"=refnum, "Acquisition Mode"=refnum, "Spectal Position"=refnum, "From"=refnum, "To"=refnum, "Integration Time"=refnum, "Accumulations"=refnum, "AutoScanning"=refnum, "Spike Removal"=refnum, "Acquisition Mode Panel"=refnum} ("LabramHR"), "Instrument Status"=w177, "Optical Spectrum Plot.Plot List"=w196, "Optical Spectrum Plot.Optical Spectrum vs Energy"=w195, "Optical Spectrum Plot.Optical Spectrum vs Wavelength"=w194, "Optical Spectrum Plot.Optical Spectrum vs Raman Shift"=w193, "Optical Spectrum Plot.Detector Temperature"=w179, "Laser"=w192, "Filter"=w191, "Hole"=w190, "Grating"=w189, "Detector"=w188, "Acquisition Mode"=w187, "Spectal Position"=w180, "From"=w186, "To"=w181, "Integration Time"=w182, "Accumulations"=w183, "AutoScanning"=w184, "Spike Removal"=w185) -> (w197:T59)
        n120 = Unbundle By Name(w201) -> ("Optical Spectrometer"=w199:refnum<queue>)
        n121 = call "Enqueue Message (Single).vi"("Message Data"=w197, "Message"="Update Refnums", "Message Queue"=w199) -> ()  [unwired: 1 in, 8 out]
      }
      frame "LabramHR - Set Laser" {
        # "Handle the change of Excitation Wavelength"
        n122 = Variant To Data(error in=w208, type=Laser."633 nm" ("NewVal"), Variant=w212) -> (data=w203:T3, error out=w207:errorcluster)
        n123 = Bundle By Name(cluster=T34 {"Laser Settings"={"Laser Wavelength"=enum."633 nm", "Neutral Density Filter"=enum."1%"}, "Spectrometer Settings"={"Confocal Hole Size (µm)"=150.0, "Grating"=1, "Detector"=enum."InGaAs Array"}, "Acquisition Settings"={"Acquisition Mode"=enum."Single Window", "Spectal Position (nm)"=480.0, "From (nm)"=632.0, "To (nm)"=1000.0, "Integration Time (s)"=3.0, "Number of Accumulations"=3, "AutoScanning"=FALSE, "Spike Removal"=FALSE}, "Path"=path ""} ("LabramHR"), "Laser Settings.Laser Wavelength"=w203) -> (w205:T34)
        n124 = Unbundle By Name(w211) -> ("Optical Spectrometer"=w210:refnum<queue>)
        n125 = call "Enqueue Message (Single).vi"("error in (no error)"=w207, "Message Data"=w205, "Message"="Set Laser", "Message Queue"=w210) -> ("error out"=w206:errorcluster)  [unwired: 7 out]
      }
      frame "LabramHR - Set Filter" {
        # "Handle the change of Neutral Density Filter"
        n126 = Variant To Data(error in=w223, type=Filter."1%" ("NewVal"), Variant=w222) -> (data=w214:T4, error out=w220:errorcluster)
        n127 = Bundle By Name(cluster=T34 {"Laser Settings"={"Laser Wavelength"=enum."633 nm", "Neutral Density Filter"=enum."1%"}, "Spectrometer Settings"={"Confocal Hole Size (µm)"=150.0, "Grating"=1, "Detector"=enum."InGaAs Array"}, "Acquisition Settings"={"Acquisition Mode"=enum."Single Window", "Spectal Position (nm)"=480.0, "From (nm)"=632.0, "To (nm)"=1000.0, "Integration Time (s)"=3.0, "Number of Accumulations"=3, "AutoScanning"=FALSE, "Spike Removal"=FALSE}, "Path"=path ""} ("LabramHR"), "Laser Settings.Neutral Density Filter"=w214) -> (w216:T34)
        n128 = Unbundle By Name(w218) -> ("Optical Spectrometer"=w221:refnum<queue>)
        n129 = call "Enqueue Message (Single).vi"("error in (no error)"=w220, "Message Data"=w216, "Message"="Set Filter", "Message Queue"=w221) -> ("error out"=w219:errorcluster)  [unwired: 7 out]
      }
      frame "LabramHR - Set Hole" {
        # "Handle the change in Confocal hole size"
        n130 = Variant To Data(error in=w234, type=150.0 ("Confocal Hole Size (µm) 2"), Variant=w233) -> (data=w226:dbl, error out=w229:errorcluster)
        n131 = Bundle By Name(cluster=T34 {"Laser Settings"={"Laser Wavelength"=enum."633 nm", "Neutral Density Filter"=enum."1%"}, "Spectrometer Settings"={"Confocal Hole Size (µm)"=150.0, "Grating"=1, "Detector"=enum."InGaAs Array"}, "Acquisition Settings"={"Acquisition Mode"=enum."Single Window", "Spectal Position (nm)"=480.0, "From (nm)"=632.0, "To (nm)"=1000.0, "Integration Time (s)"=3.0, "Number of Accumulations"=3, "AutoScanning"=FALSE, "Spike Removal"=FALSE}, "Path"=path ""} ("LabramHR"), "Spectrometer Settings.Confocal Hole Size (µm)"=w226) -> (w225:T34)
        n132 = Unbundle By Name(w227) -> ("Optical Spectrometer"=w231:refnum<queue>)
        n133 = call "Enqueue Message (Single).vi"("error in (no error)"=w229, "Message Data"=w225, "Message"="Set Hole", "Message Queue"=w231) -> ("error out"=w230:errorcluster)  [unwired: 7 out]
      }
      frame "LabramHR - Set Grating" {
        w236 = T6 1 items=["1800 l/mm", "150 l/mm"] ("NewVal")
        # "Handle the change of grating"
        n134 = Variant To Data(error in=w245, type=w236, Variant=w244) -> (data=w238:T6, error out=w241:errorcluster)
        n135 = Bundle By Name(cluster=T34 {"Laser Settings"={"Laser Wavelength"=enum."633 nm", "Neutral Density Filter"=enum."1%"}, "Spectrometer Settings"={"Confocal Hole Size (µm)"=150.0, "Grating"=1, "Detector"=enum."InGaAs Array"}, "Acquisition Settings"={"Acquisition Mode"=enum."Single Window", "Spectal Position (nm)"=480.0, "From (nm)"=632.0, "To (nm)"=1000.0, "Integration Time (s)"=3.0, "Number of Accumulations"=3, "AutoScanning"=FALSE, "Spike Removal"=FALSE}, "Path"=path ""} ("LabramHR"), "Spectrometer Settings.Grating"=w238) -> (w237:T34)
        n136 = Unbundle By Name(w240) -> ("Optical Spectrometer"=w243:refnum<queue>)
        n137 = call "Enqueue Message (Single).vi"("error in (no error)"=w241, "Message Data"=w237, "Message"="Set Grating", "Message Queue"=w243) -> ("error out"=w242:errorcluster)  [unwired: 7 out]
      }
      frame "LabramHR - Set Detector" {
        # "Handle the change of grating"
        n138 = Variant To Data(error in=w256, type=Detector."Silicon CCD" ("NewVal"), Variant=w255) -> (data=w249:T7, error out=w252:errorcluster)
        n139 = Bundle By Name(cluster=T34 {"Laser Settings"={"Laser Wavelength"=enum."633 nm", "Neutral Density Filter"=enum."1%"}, "Spectrometer Settings"={"Confocal Hole Size (µm)"=150.0, "Grating"=1, "Detector"=enum."InGaAs Array"}, "Acquisition Settings"={"Acquisition Mode"=enum."Single Window", "Spectal Position (nm)"=480.0, "From (nm)"=632.0, "To (nm)"=1000.0, "Integration Time (s)"=3.0, "Number of Accumulations"=3, "AutoScanning"=FALSE, "Spike Removal"=FALSE}, "Path"=path ""} ("LabramHR"), "Spectrometer Settings.Detector"=w249) -> (w248:T34)
        n140 = Unbundle By Name(w251) -> ("Optical Spectrometer"=w254:refnum<queue>)
        n141 = call "Enqueue Message (Single).vi"("error in (no error)"=w252, "Message Data"=w248, "Message"="Set Detector", "Message Queue"=w254) -> ("error out"=w253:errorcluster)  [unwired: 7 out]
      }
      frame "LabramHR - Set Spectal Position" {
        # "Handle the change of Spetrometer position"
        n142 = Variant To Data(error in=w267, type=480.0 ("Spectal Position (nm) 2"), Variant=w266) -> (data=w259:dbl, error out=w261:errorcluster)
        n143 = Bundle By Name(cluster=T34 {"Laser Settings"={"Laser Wavelength"=enum."633 nm", "Neutral Density Filter"=enum."1%"}, "Spectrometer Settings"={"Confocal Hole Size (µm)"=150.0, "Grating"=1, "Detector"=enum."InGaAs Array"}, "Acquisition Settings"={"Acquisition Mode"=enum."Single Window", "Spectal Position (nm)"=480.0, "From (nm)"=632.0, "To (nm)"=1000.0, "Integration Time (s)"=3.0, "Number of Accumulations"=3, "AutoScanning"=FALSE, "Spike Removal"=FALSE}, "Path"=path ""} ("LabramHR"), "Acquisition Settings.Spectal Position (nm)"=w259) -> (w258:T34)
        n144 = Unbundle By Name(w260) -> ("Optical Spectrometer"=w264:refnum<queue>)
        n145 = call "Enqueue Message (Single).vi"("error in (no error)"=w261, "Message Data"=w258, "Message"="Set Spectal Position", "Message Queue"=w264) -> ("error out"=w263:errorcluster)  [unwired: 7 out]
      }
      frame "LabramHR - Set Acquisition Settings" {
        # "Handle the change of integration time"
        n146 = Variant To Data(error in=w278, type=T8 {"Acquisition Mode"=enum."Single Window", "Spectal Position (nm)"=480.0, "From (nm)"=632.0, "To (nm)"=1000.0, "Integration Time (s)"=3.0, "Number of Accumulations"=3, "AutoScanning"=FALSE, "Spike Removal"=FALSE} ("Acquisition Settings 2"), Variant=w277) -> (data=w271:T8, error out=w275:errorcluster)
        n147 = Bundle By Name(cluster=T34 {"Laser Settings"={"Laser Wavelength"=enum."633 nm", "Neutral Density Filter"=enum."1%"}, "Spectrometer Settings"={"Confocal Hole Size (µm)"=150.0, "Grating"=1, "Detector"=enum."InGaAs Array"}, "Acquisition Settings"={"Acquisition Mode"=enum."Single Window", "Spectal Position (nm)"=480.0, "From (nm)"=632.0, "To (nm)"=1000.0, "Integration Time (s)"=3.0, "Number of Accumulations"=3, "AutoScanning"=FALSE, "Spike Removal"=FALSE}, "Path"=path ""} ("LabramHR"), "Acquisition Settings"=w271) -> (w270:T34)
        n148 = Unbundle By Name(w272) -> ("Optical Spectrometer"=w273:refnum<queue>)
        n149 = call "Enqueue Message (Single).vi"("error in (no error)"=w275, "Message Data"=w270, "Message"="Set Acquisition Settings", "Message Queue"=w273) -> ("error out"=w276:errorcluster)  [unwired: 7 out]
      }
      frame "LabramHR - Acquire Spectrum" {
        n150 = Unbundle By Name(w280) -> ("Optical Spectrometer"=w281:refnum<queue>)
        n151 = call "Enqueue Message (Single).vi"("error in (no error)"=w282, "Message"="Acquire Spectrum", "Message Queue"=w281) -> ("error out"=w279:errorcluster)  [unwired: 1 in, 7 out]
      }
      frame "LabramHR - Save Spectrum" {
        n152 = Unbundle By Name(w285) -> ("Optical Spectrometer"=w286:refnum<queue>)
        n153 = call "Enqueue Message (Single).vi"("error in (no error)"=w287, "Message"="Save Optical Spectrum", "Message Queue"=w286) -> ("error out"=w284:errorcluster)  [unwired: 1 in, 7 out]
      }
      frame "Instrument Sequence - Pause Sequence" {
        n154 = Unbundle By Name(w293) -> ("Instrument Sequence"=w292:refnum<queue>)
        n155 = call "Enqueue Message (Single).vi"("error in (no error)"=w289, "Message"="Pause Sequence", "Message Queue"=w292) -> ("error out"=w291:errorcluster)  [unwired: 1 in, 7 out]
      }
      frame "----- Save Data Events -----" {
        # "Save Data Events"
      }
    }
    n156 = call "Message Handling Loop.vi"("error in (no error)"=w36, "Message Queue"=w34) -> ("dup error in"=w35:errorcluster)  [unwired: 9 out]
  }
  n157 = while "Event Handling Loop" {
    tunnel: w22 -> [w301]
    tunnel: [w300] -> w21
    tunnel: w20 -> [w298]
    tunnel: [w296] -> w19
    stop <- w295 stop-if-true
    n158 = event shown="[2] \"Exit\": Value Change" {
      selector: w301 -> [_ _ _ _ _ _ _ _ _ _ _ _ _]
      dyn-events: [_ _ _ _ _ _ _ _ _ _ _ _ _] -> w296
      timeout: _ -> [_ _ _ _ _ _ _ _ _ _ _ _ _]
      tunnel: [w303 _ w311 _ w321 w329 w334 w339 w344 w349 w354 w355 w361] -> w299
      tunnel: w298 -> [w306 w308 w313 w318 w323 w327 w332 w337 w342 w347 w352 w357 w360]
      tunnel: [w302 w308 w312 w318 w322 w328 w333 w338 w343 w348 w353 w356 w362] -> w297
      tunnel: [_ _ _ TRUE ("Priority Message? (F)") _ _ _ _ _ _ _ _ _] -> w295
      event Panel Close? {
        # "Send the \"Confirm Quit\" message if the user closes the panel of the VI. Discard the event so the \"Confirm Quit\" message has a chance to run."
        n159 = event-data() -> ()  [unwired: 2 out]
        n160 = call "Enqueue Message (Single).vi"("Priority Message? (F)"=TRUE, "Message"="Initiate Exit", "Message Queue"=w306) -> ("error out"=w303:errorcluster, "dup Message Queue"=w302:refnum<queue>)  [unwired: 2 in, 5 out]
        n161 = event-data("Discard?"=TRUE) -> ()  [unwired: 1 in, 1 out]
      }
      event Application Instance Close {
        # "#CodeRecommended - When a project closes, all VIs within that project are aborted and leave memory. However, any code placed in this event frame is guaranteed to run to completion, so add any cleanup code that absolutely must happen here."
        n162 = event-data() -> ()  [unwired: 2 out]
      }
      event "Exit": Value Change {
        n163 = event-data() -> ()  [unwired: 2 out]
        n164 = call "Enqueue Message (Single).vi"("Priority Message? (F)"=TRUE, "Message"="Initiate Exit", "Message Queue"=w313) -> ("error out"=w311:errorcluster, "dup Message Queue"=w312:refnum<queue>)  [unwired: 2 in, 5 out]
      }
      event User Event {
        n165 = event-data() -> ()  [unwired: 2 out]
        n166 = call "Status String.vi"("Message"="Program Terminated" ("Display <Replace Me>")) -> ("Status String"=w314:string)
        n167 = property on="Status Log" class="Str"() -> ("Value"=w316:string)  [unwired: 2 in, 2 out]
        n168 = Concatenate Strings(w314, w316) -> (w317:string)
        n169 = property on="Status Log" class="Str"("Value"=w317) -> ()  [unwired: 2 in, 2 out]
      }
      event Value Change {
        n170 = event-data() -> ("NewVal"=w320:T3)  [unwired: 1 out]
        n171 = call "Enqueue Message (Single).vi"("Message Data"=w320, "Message"="LabramHR - Set Laser", "Message Queue"=w323) -> ("error out"=w321:errorcluster, "dup Message Queue"=w322:refnum<queue>)  [unwired: 1 in, 6 out]
      }
      event Value Change {
        n172 = event-data() -> ("NewVal"=w325:T4)  [unwired: 1 out]
        n173 = call "Enqueue Message (Single).vi"("Message Data"=w325, "Message"="LabramHR - Set Filter", "Message Queue"=w327) -> ("error out"=w329:errorcluster, "dup Message Queue"=w328:refnum<queue>)  [unwired: 1 in, 6 out]
      }
      event Value Change {
        n174 = event-data() -> ("NewVal"=w330:dbl)  [unwired: 1 out]
        n175 = call "Enqueue Message (Single).vi"("Message Data"=w330, "Message"="LabramHR - Set Hole", "Message Queue"=w332) -> ("error out"=w334:errorcluster, "dup Message Queue"=w333:refnum<queue>)  [unwired: 1 in, 6 out]
      }
      event Value Change {
        n176 = event-data() -> ("NewVal"=w335:T6)  [unwired: 1 out]
        n177 = call "Enqueue Message (Single).vi"("Message Data"=w335, "Message"="LabramHR - Set Grating", "Message Queue"=w337) -> ("error out"=w339:errorcluster, "dup Message Queue"=w338:refnum<queue>)  [unwired: 1 in, 6 out]
      }
      event Value Change {
        n178 = event-data() -> ("NewVal"=w340:T7)  [unwired: 1 out]
        n179 = call "Enqueue Message (Single).vi"("Message Data"=w340, "Message"="LabramHR - Set Detector", "Message Queue"=w342) -> ("error out"=w344:errorcluster, "dup Message Queue"=w343:refnum<queue>)  [unwired: 1 in, 6 out]
      }
      event Value Change {
        n180 = event-data() -> ("NewVal"=w345:dbl)  [unwired: 1 out]
        n181 = call "Enqueue Message (Single).vi"("Message Data"=w345, "Message"="LabramHR - Set Spectal Position", "Message Queue"=w347) -> ("error out"=w349:errorcluster, "dup Message Queue"=w348:refnum<queue>)  [unwired: 1 in, 6 out]
      }
      event Value Change {
        n182 = event-data() -> ()  [unwired: 3 out]
        n183 = call "Enqueue Message (Single).vi"("Message Data"="Acquisition Settings", "Message"="LabramHR - Set Acquisition Settings", "Message Queue"=w352) -> ("error out"=w354:errorcluster, "dup Message Queue"=w353:refnum<queue>)  [unwired: 1 in, 6 out]
      }
      event "Optical Spectrometer - Measure": Value Change {
        n184 = event-data() -> ()  [unwired: 3 out]
        n185 = call "Enqueue Message (Single).vi"("Message"="LabramHR - Acquire Spectrum", "Message Queue"=w357) -> ("error out"=w355:errorcluster, "dup Message Queue"=w356:refnum<queue>)  [unwired: 2 in, 6 out]
      }
      event "Optical Spectrometer - Save Measurement": Value Change {
        n186 = event-data() -> ()  [unwired: 3 out]
        n187 = call "Enqueue Message (Single).vi"("Message"="LabramHR - Save Spectrum", "Message Queue"=w360) -> ("error out"=w361:errorcluster, "dup Message Queue"=w362:refnum<queue>)  [unwired: 2 in, 6 out]
      }
    }
    n188 = call "Event Handling Loop.vi"("error in (no error)"=w299, "Message Queue"=w297) -> ("dup error in"=w300:errorcluster)  [unwired: 9 out]
  }
  n189 = Unregister For Events(event registration refnum=w19, error in=w21) -> (error out=w5:errorcluster)
  n190 = Merge Errors(w5, w4, w3, w1) -> (w14:errorcluster)
  n191 = call "Close Notifiers.vi"("error in"=w14, "Notifiers"=w6) -> ("error out"=w13:errorcluster)  [unwired: 9 out]
  n192 = call "Destroy User Event - Stop.vi"("error in (no error)"=w13, "User Event - Stop"=w15) -> ("error out"=w18:errorcluster)  [unwired: 9 out]
  n193 = property class="App"(error in=w18) -> (error out=w16:errorcluster, "App.Kind"=w17:T61)  [unwired: 1 in, 1 out]
  n194 = case shown="\"Development System\"" w17 {
    tunnel: w16 -> [w363 w364 _ _ _ _ _]
    frame "invalid app kind", Default {
      n195 = call <vilib>:"Simple Error Handler.vi"("error in (no error)"=w363) -> ()  [unwired: 1 in, 8 out]
    }
    frame "Development System" {
      n196 = call <vilib>:"Simple Error Handler.vi"("error in (no error)"=w364) -> ()  [unwired: 1 in, 8 out]
    }
    frame "Run Time System" {
      n197 = Quit LabVIEW() -> ()  [unwired: 1 out]
    }
    frame "Student Edition" {
    }
    frame "Embedded LabVIEW" {
    }
    frame "Evaluation" {
    }
    frame "Custom" {
    }
  }
